vi "Save Grid to File.vi"(8 "error in (no error)":errorcluster, 10 "file path":path, 11 "occupancy grid":dbl[][](array[numeric])) -> (0 "error out":errorcluster)   [LabVIEW 2017]
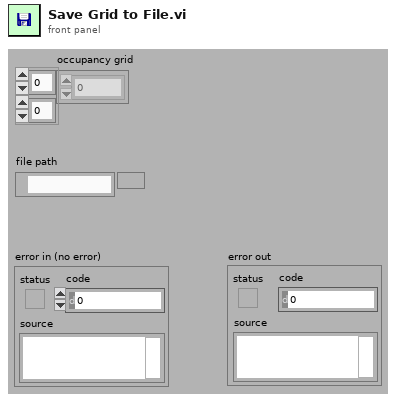
[diagram p1: front panel]
types:
  T1 = enum16{"open", "replace", "create", "open or create", "replace or create", "replace or create with confirmation"}
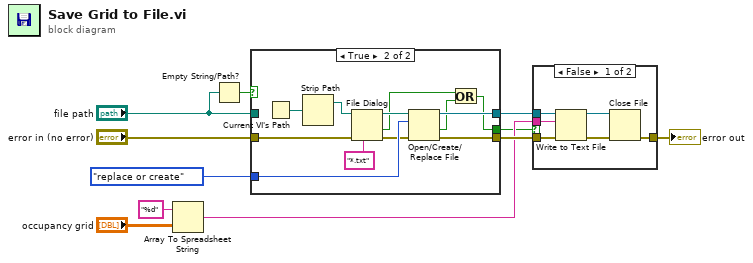
[diagram p0: block diagram]
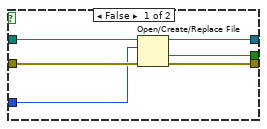
[diagram p3: hidden frame]
diagram:
  n1 = Array To Spreadsheet String(array="occupancy grid", 3:"%d" ("format string")) -> (spreadsheet string=w7:string)  [unwired: 1 in]
  n2 = Empty String/Path?(string/path="file path") -> (empty?=w2:bool)
  n3 = case shown="True" w2 {
    tunnel: [w17 w29] -> w9
    tunnel: [w16 w28] -> w8
    tunnel: "error in (no error)" -> [w15 w23]
    tunnel: T1."replace or create" ("operation (0:open)") -> [w14 w27]
    tunnel: "file path" -> [w13 _]
    tunnel: [w12 w19] -> w1
    frame False {
      n4 = Open/Create/Replace File(file path (use dialog)=w13, error in=w15, operation (0:open)=w14) -> (refnum out=w17:refnum<file>, cancelled=w12:bool, error out=w16:errorcluster)  [unwired: 3 in]
    }
    frame True {
      n5 = Current VI's Path() -> (path=w24:path)
      n6 = Strip Path(path=w24) -> (stripped path=w25:path)  [unwired: 1 out]
      n7 = File Dialog(6:"*.txt" ("pattern (all files)"), 8:w23, 11:w25) -> (0:w22:errorcluster, 1:w18:bool, 3:w21:path)  [unwired: 4 in, 1 out]
      n8 = Open/Create/Replace File(file path (use dialog)=w21, error in=w22, operation (0:open)=w27) -> (refnum out=w29:refnum<file>, cancelled=w20:bool, error out=w28:errorcluster)  [unwired: 3 in]
      n9 = Or(x=w18, y=w20) -> (x .or. y?=w19:bool)
    }
  }
  n10 = case shown="False" w1 {
    tunnel: w9 -> [w35 _]
    tunnel: w8 -> [w34 _]
    tunnel: w7 -> [w33 _]
    tunnel: [w30 _] -> w6
    frame False {
      n11 = Write to Text File(file (use dialog)=w35, text=w33, error in=w34) -> (refnum out=w32:refnum<file>, error out=w31:errorcluster)  [unwired: 1 in, 1 out]
      n12 = Close File(refnum=w32, error in=w31) -> (error out=w30:errorcluster)  [unwired: 1 out]
    }
    frame True {
    }
  }
  "error out" <- w6
